vi "temp_sensor.vi"() -> ()   [LabVIEW 2018]
uses:
  <vilib>/DAQmx/read.llb/DAQmx Read (Analog DBL 1Chan 1Samp).vi
  <vilib>/DAQmx/miscellaneous.llb/DAQmx Fill In Error Info.vi
panel:
  out "Thermometer":dbl(slide) scale=0.0..100.0
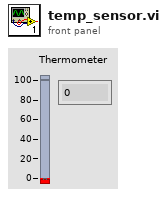
[diagram p1: front panel]
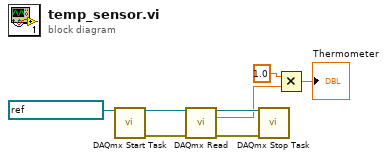
[diagram p0: block diagram]
diagram:
  n1 = call <vilib>:"DAQmx Start Task.vi"("task/channels in"=refnum<k21> "temp_sensor") -> ("task out"=w5:refnum<k21>, "error out"=w7:errorcluster)  [unwired: 13 in]
  n2 = call-poly <vilib>:"DAQmx Read.vi"("task/channels in"=w5, "error in"=w7) -> ("task out"=w6:refnum<k21>, "data"=w3:dbl, "error out"=w8:errorcluster)  [unwired: 11 in]
  n3 = call <vilib>:"DAQmx Stop Task.vi"("task/channels in"=w6, "error in"=w8) -> ()  [unwired: 12 in, 2 out]
  n4 = Multiply(x=1.0, y=w3) -> (x*y=→"Thermometer":dbl)
